vi "hw9p7_hickey.vi"() -> ()   [LabVIEW 2014]
panel:
  in  "Guess":dbl
  in  "Enter Guess":bool
  out "Message":string
  # "Top shift register: the next case of the case statement"
  # "Lower shift register: the guess"
  # "State 0 asks for the number and goes to state 1"
  # "State 1 takes your guess and goes to state 2"
  # "State 2 checks if your guess is correct and goes to \nstate 3 or 4 accordingly"
  # "State 3 tells you if your guess is too high or two low\nand goes to state 1 so you can guess again"
  # "State 4 tells you that you are right and stops the program"
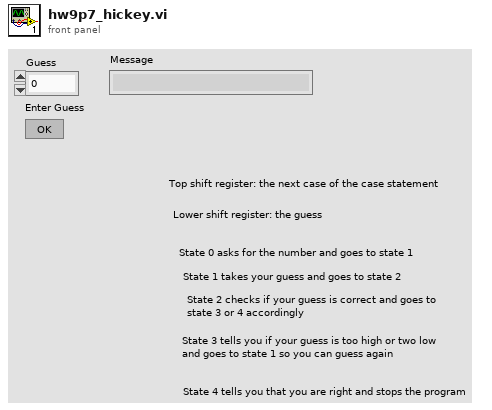
[diagram p1: front panel]
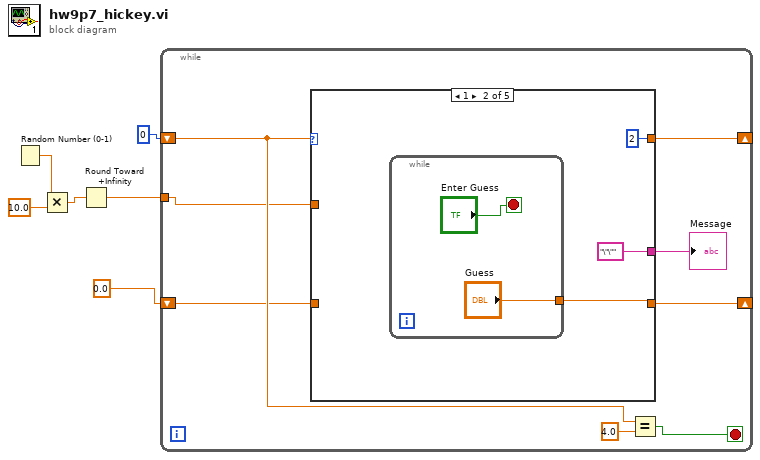
[diagram p0: block diagram]
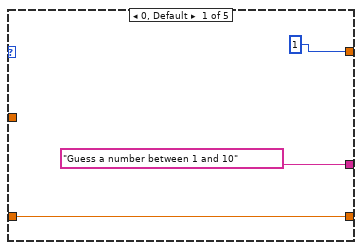
[diagram p2: hidden frame]
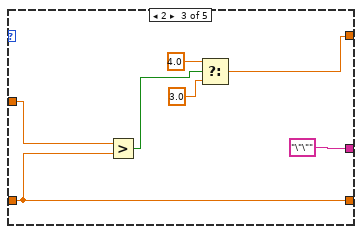
[diagram p3: hidden frame]
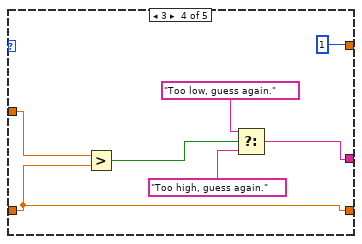
[diagram p4: hidden frame]
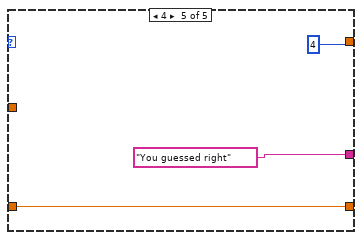
[diagram p5: hidden frame]
diagram:
  n1 = Random Number (0-1)() -> (number: 0 to 1=w4:dbl)
  n2 = Multiply(x=w4, y=10.0) -> (x*y=w3:dbl)
  n3 = Round Toward +Infinity(x=w3) -> (ceil(x): smallest int >= x=w2:dbl)
  n4 = while {
    shift-right: [w9] -> _
    shift-left: 0 -> [w13]
    tunnel: w2 -> [w11]
    shift-right: [w7] -> _
    shift-left: 0.0 ("y") -> [w10]
    stop <- w12 stop-if-true
    n5 = case shown="1" w13 {
      tunnel: w11 -> [_ _ w29 w35 _]
      tunnel: w10 -> [w15 _ w28 w34 w39]
      tunnel: [1 2 w24 1 4] -> w9
      tunnel: ["Guess a number between 1 and 10" ("Message") "\"\"" ("Message") "\"\"" ("Message") w32 "You guessed right" ("Message")] -> w8
      tunnel: [w15 w20 w28 w34 w39] -> w7
      frame 0, Default {
      }
      frame 1 {
        n6 = while {
          tunnel: ["Guess"] -> w20
          stop <- "Enter Guess" stop-if-true
        }
      }
      frame 2 {
        n7 = Greater?(x=w29, y=w28) -> (0:w25:bool)
        n8 = Select(t=4.0, s=w25, f=3.0 ("t")) -> (s? t:f=w24:dbl)
      }
      frame 3 {
        n9 = Greater?(x=w35, y=w34) -> (0:w33:bool)
        n10 = Select(t="Too low, guess again." ("Message"), s=w33, f="Too high, guess again." ("Message")) -> (s? t:f=w32:string)
      }
      frame 4 {
      }
    }
    "Message" <- w8
    n11 = Equal?(x=w13, y=4.0) -> (x = y?=w12:bool)
  }
